vi "wa32 WriteFile.vi"(8 "error in":errorcluster, 9 "string data (empty)":string, 10 "data (empty)":u8[](array[numeric]), 11 "handle":i32) -> (0 "error out":errorcluster, 2 "written bytes":u32, 3 "handle out":i32)   [LabVIEW 2018]
doc: "WinAPI WriteFile() wrapper. For writting opened handle (files, devices, pipes, ...)."
uses:
  <vilib>/Utility/error.llb/Error Cluster From Error Code.vi
  <vilib>/ErrorRing/Error Ring.xnode
  kernel32.dll
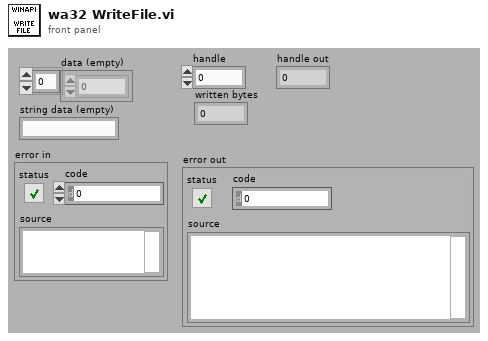
[diagram p1: front panel]
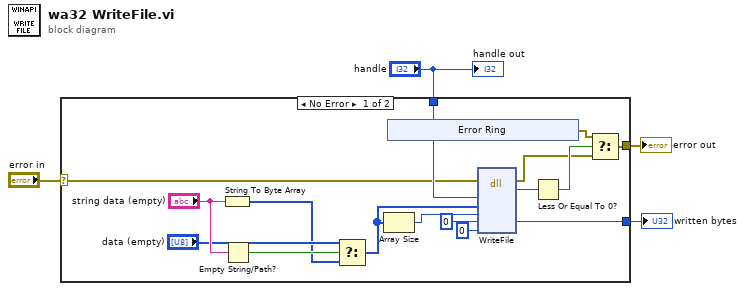
[diagram p0: block diagram]
diagram:
  n1 = case shown="No Error" "error in" {
    selector: "error in" -> [w6 w26]
    tunnel: [w17 _] -> w4
    tunnel: [w9 w26] -> w3
    tunnel: "handle" -> [w7 _]
    frame No Error {
      n2 = String To Byte Array(string="string data (empty)") -> (unsigned byte array=w5:u8[])
      n3 = Empty String/Path?(string/path="string data (empty)") -> (empty?=w15:bool)
      n4 = Select(t="data (empty)", s=w15, f=w5) -> (s? t:f=w13:u8[])
      n5 = Array Size(array=w13) -> (size(s)=w18:i32)
      n6 = xnode "Error Ring"() -> ("error out"=w8:errorcluster)
      n7 = dll-call lib="kernel32.dll" fn="WriteFile"(error in=w6, "handle"=w7, "data"=w13, "toWrite"=w18, "written"=u32 0, "overlapped"=0) -> (error out=w10:errorcluster, "errout"=w12:i32, "written"=w17:u32)  [unwired: 6 in, 1 out]
      n8 = Less Or Equal To 0?(x=w12) -> (x <= 0?=w11:bool)
      n9 = Select(t=w8, s=w11, f=w10) -> (s? t:f=w9:errorcluster)
    }
    frame Error {
    }
  }
  "error out" <- w3
  "written bytes" <- w4
  "handle out" <- "handle"
